vi "test Last Ack_Error_Returns Context Actor.vi"() -> ()   [LabVIEW 2020]
uses:
  Test Harness/Context Actor with Error/Context Actor with Error.lvclass
  C:/Program Files (x86)/National Instruments/LabVIEW 2020/vi.lib/ActorFramework/Actor/Actor.lvclass
  <vilib>/ActorFramework/LastAck/Last Ack.lvclass
  <vilib>/ActorFramework/Message Queue/Message Queue.lvclass/Message Queue.ctl
  <vilib>/ActorFramework/Message Dequeuer/Message Dequeuer.lvclass/Message Dequeuer.ctl
  <vilib>/ActorFramework/LastAck/Last Ack.lvclass/Last Ack.ctl
  <vilib>/ActorFramework/Message Enqueuer/Message Enqueuer.lvclass/Message Enqueuer.ctl
  <vilib>/ActorFramework/Message Enqueuer/Enqueue.vi
  <vilib>/ActorFramework/Stop Msg/Stop Msg.lvclass
  C:/Program Files (x86)/National Instruments/LabVIEW 2020/vi.lib/ActorFramework/Message/Message.lvclass
  <vilib>/ActorFramework/Message Priority Queue/Priority Dequeue.vi
  <vilib>/ActorFramework/Message Priority Queue/Priority Enqueue.vi
  <vilib>/addons/_JKI Toolkits/Caraya/classes/Assert/Assert Not Error.vi
  <vilib>/addons/_JKI Toolkits/Caraya/classes/Test/Test.lvclass
  <vilib>/addons/_JKI Toolkits/Caraya/classes/Assert/Assert.lvclass
  <vilib>/ActorFramework/Actor/Actor.lvclass
  <vilib>/ActorFramework/Message Queue/Message Queue.lvclass
  <vilib>/ActorFramework/Message Dequeuer/Message Dequeuer.lvclass
panel:
  out "error out":errorcluster
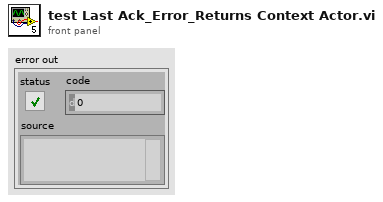
[diagram p1: front panel]
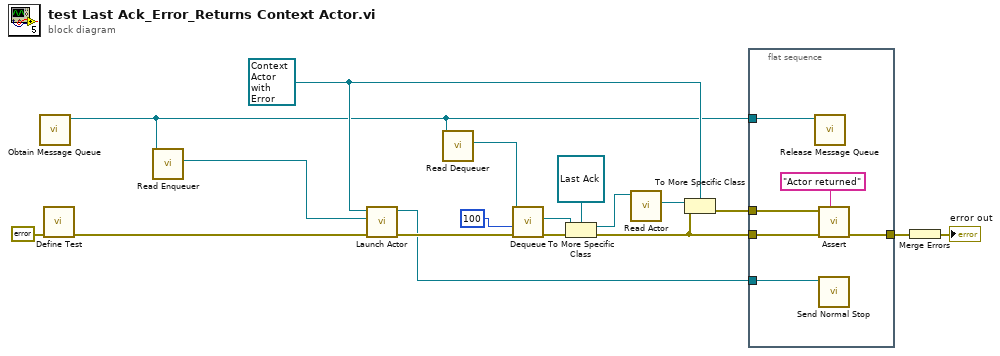
[diagram p0: block diagram]
diagram:
  w7 = refnum<class "Context Actor with Error.lvclass"> refnum ("Context Actor with Error.lvclass")
  n1 = call <vilib>:"Obtain Message Queue.vi"() -> ("Message Queue"=w4:refnum<class "Message Queue.lvclass">)  [unwired: 10 in, 1 out]
  n2 = call <vilib>:"Define Test.vi"("error in (no error)"=errorcluster {"status"=FALSE, "code"=0, "source"=""}) -> ("error out"=w16:errorcluster)  [unwired: 9 in, 1 out]
  n3 = call <vilib>:"Read Enqueuer.vi"("Message Queue"=w4) -> ("Message Enqueuer"=w14:refnum<class "Message Enqueuer.lvclass">)  [unwired: 10 in]
  n4 = call <vilib>:"Launch Actor.vi"("error in (no error)"=w16, "Actor-to-Caller Enqueuer"=w14, "Actor"=w7) -> ("error out"=w15:errorcluster, "Caller-To-Actor Enqueuer"=w3:refnum<class "Message Enqueuer.lvclass">)  [unwired: 7 in]
  n5 = call <vilib>:"Read Dequeuer.vi"("Message Queue"=w4) -> ("Message Dequeuer"=w12:refnum<class "Message Dequeuer.lvclass">)  [unwired: 10 in]
  n6 = call <vilib>:"Dequeue.vi"("error in (no error)"=w15, "timeout in ms (-1)"=100, "Message Dequeuer in"=w12) -> ("error out"=w13:errorcluster, "Message"=w1:refnum<class "Message.lvclass">)  [unwired: 4 in, 3 out]
  n7 = To More Specific Class(target class=refnum<class "Last Ack.lvclass"> refnum ("Last Ack"), reference=w1, error in=w13) -> (specific class reference=w9:refnum<class "Last Ack.lvclass">, error out=w6:errorcluster)
  n8 = call <vilib>:"Read Actor.vi"("Last Ack"=w9) -> ("Actor"=w8:refnum<class "Actor.lvclass">)  [unwired: 10 in]
  n9 = To More Specific Class(target class=w7, reference=w8, error in=w6) -> (error out=w5:errorcluster)  [unwired: 1 out]
  n10 = flat-sequence {
    tunnel: [w23] -> w18
    tunnel: w6 -> [w22]
    tunnel: w5 -> [w21]
    tunnel: w4 -> [w20]
    tunnel: w3 -> [w19]
    frame #0 {
      n11 = call <vilib>:"Release Message Queue.vi"("Message Queue"=w20) -> ()  [unwired: 9 in, 2 out]
      n12 = call-poly <vilib>:"Assert.vi"("Label"="Actor returned" ("Label (VI Title)"), "error in (no error)"=w22, "Not Error?"=w21) -> ("error out"=w23:errorcluster)  [unwired: 7 in, 1 out]
      n13 = call <vilib>:"Send Normal Stop.vi"("Message Enqueuer"=w19) -> ()  [unwired: 10 in, 1 out]
    }
  }
  n14 = Merge Errors(w18) -> (→"error out":errorcluster)
